vi "AMC e.bloxx Read Value - Boolean.vi"(8 "error in (no error)":errorcluster, 9 "Channel":i32, 10 "Module Address":i32, 11 "VISA Resource Name":refnum<visa-resource-name>) -> (0 "error out":errorcluster, 2 "Value":bool, 3 "VISA Resource Name out":refnum<visa-resource-name>)   [LabVIEW 2013]
doc: "<B>AMC - Analytik & Messtechnik GmbH Chemnitz</B>\n\nLabVIEW Drivers for e.bloxx series from Gantner Instruments\n\nThis VI reads a value from a variable specified by <B>Module Address</B> and <B>Variable</B> (starts counting with 0)."
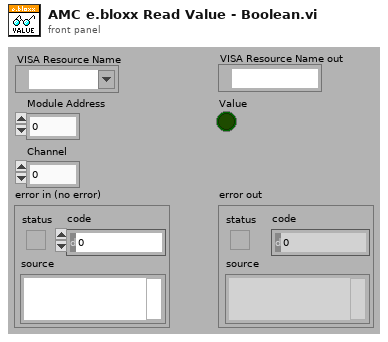
[diagram p1: front panel]
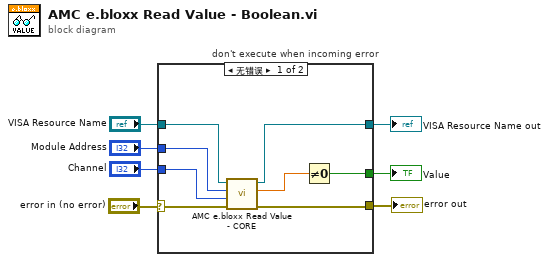
[diagram p0: block diagram]
diagram:
  n1 = case "don't execute when incoming error" shown="无错误" "error in (no error)" {
    selector: "error in (no error)" -> [w15 w17]
    tunnel: [w11 w17] -> w6
    tunnel: "VISA Resource Name" -> [w12 w16]
    tunnel: "Module Address" -> [w14 _]
    tunnel: [w10 w16] -> w3
    tunnel: "Channel" -> [w13 _]
    tunnel: [w8 _] -> w1
    frame No Error {
      n2 = call "AMC e.bloxx Read Value - CORE.vi"("error in (no error)"=w15, "Channel"=w13, "Module Address"=w14, "VISA Resource Name"=w12) -> ("error out"=w11:errorcluster, "Value"=w9:dbl, "VISA Resource Name out"=w10:refnum<visa-resource-name>)  [unwired: 5 in]
      n3 = Not Equal To 0?(x=w9) -> (x != 0?=w8:bool)
    }
    frame Error {
    }
  }
  "error out" <- w6
  "VISA Resource Name out" <- w3
  "Value" <- w1
